vi "typedef test.vi"() -> ()   [LabVIEW 2023]
uses:
  JSON Schema Generator.lvlib
  <vilib>/JDP Science/JSONtext/JSONtext.lvlib
  Example/Example Cluster 1.ctl
panel:
  out "error out":errorcluster
  in  "Example Cluster":T1={"ProductId"=1, "productName"="A green door", "price"=12.5, "tags"=["home", "green"], "ProductNumber"=1, "ProductInfoInternal"={"ProductState"=enum."Active", "State Info"={"Date"="", "Time"=0.0}}, "Product History"=[]}
  out "<JSON>":string
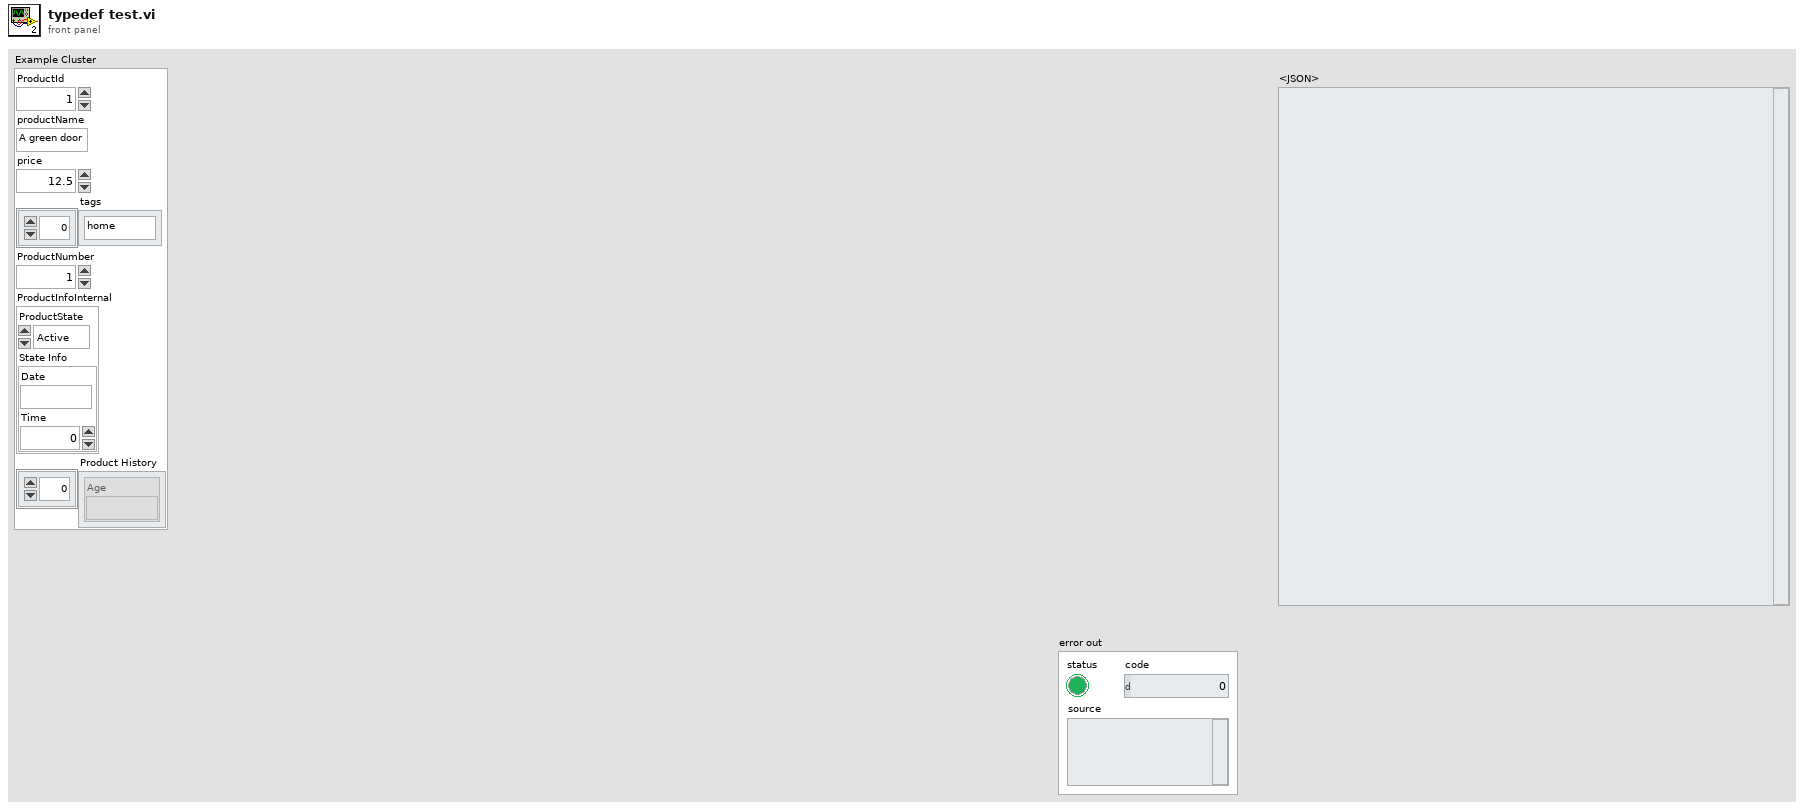
[diagram p1: front panel]
types:
  T1 = typedef "Example Cluster 1.ctl" = cluster{"ProductId":i32, "productName":string, "price":dbl, "tags":string[], "ProductNumber":i32, "ProductInfoInternal":cluster{"ProductState":enum16{"Active", "InActive"}, "State Info":cluster{"Date":string, "Time":dbl}}, "Product History":cluster{"Age":string}[]}
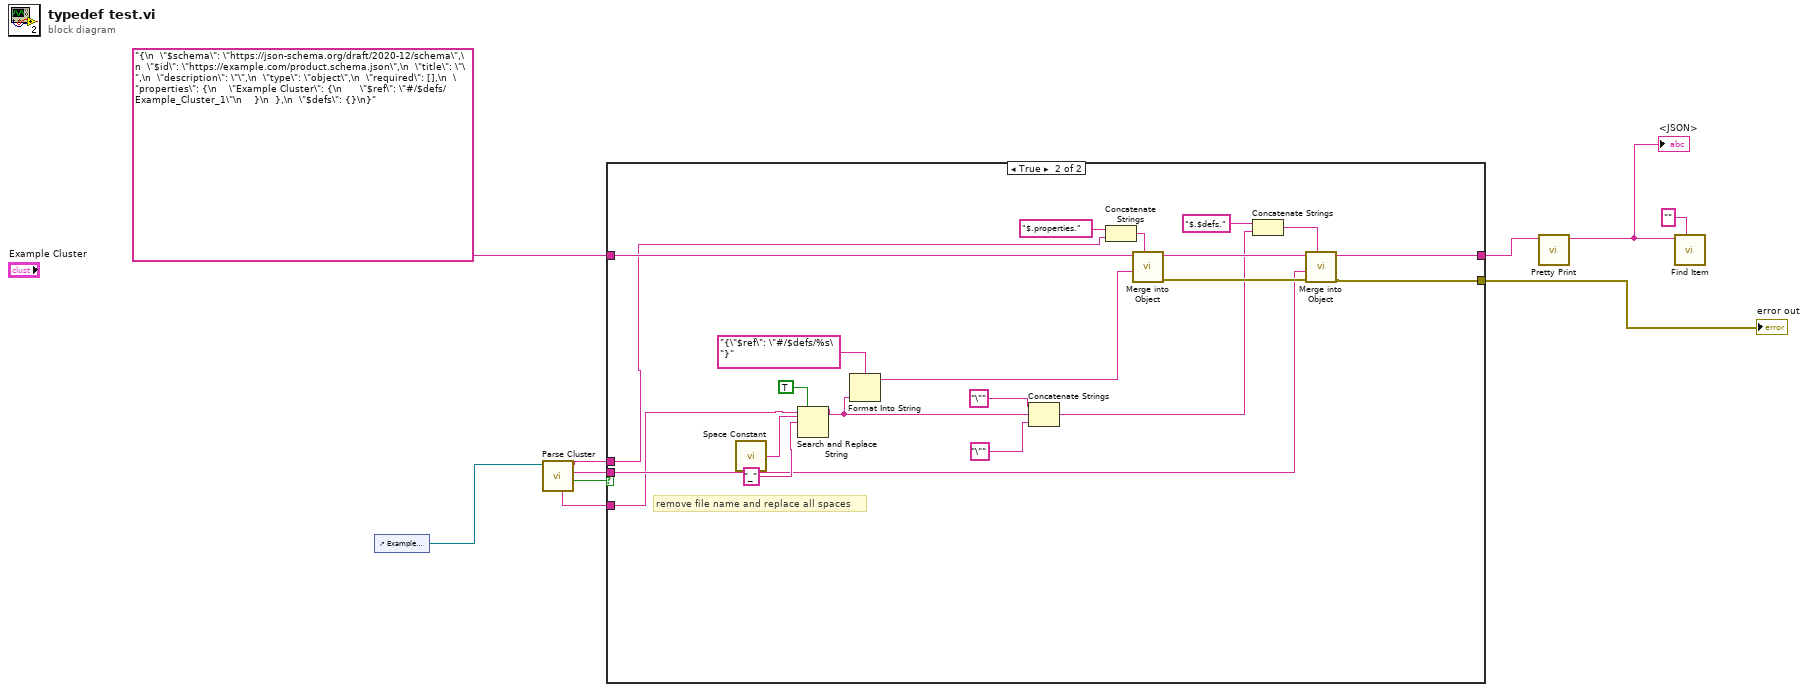
[diagram p0: block diagram]
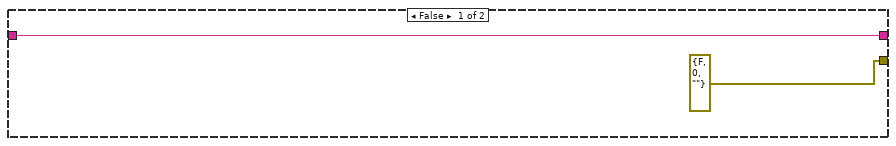
[diagram p2: hidden frame]
diagram:
  n1 = control-ref of="Example Cluster"() -> (w7:refnum<vi>)
  n2 = call "Parse Cluster.vi"("Cluster Refnum In"=w7) -> ("Typedef?"=w3:bool, "JSON ObjectSchema out"=w6:string, "JSON Object Name"=w1:string, "Typedef Name"=w2:string)  [unwired: 6 in, 1 out]
  n3 = case shown="True" w3 {
    tunnel: [w11 w29] -> w10
    tunnel: [errorcluster {"status"=FALSE, "code"=0, "source"=""} ("error out") w24] -> w9
    tunnel: "{\n  \"$schema\": \"https://json-schema.org/draft/2020-12/schema\",\n  \"$id\": \"https://example.com/product.schema.json\",\n  \"title\": \"\",\n  \"description\": \"\",\n  \"type\": \"object\",\n  \"required\": [],\n  \"properties\": {\n    \"Example Cluster\": {\n      \"$ref\": \"#/$defs/Example_Cluster_1\"\n    }\n  },\n  \"$defs\": {}\n}" ("JSON") -> [w11 w19]
    tunnel: w6 -> [_ w18]
    tunnel: w2 -> [_ w14]
    tunnel: w1 -> [_ w13]
    frame False {
    }
    frame True {
      # "remove file name and replace all spaces"
      n4 = call <vilib>:"Space Constant.vi"() -> ("String"=w21:string)
      n5 = Search and Replace String(replace all?=TRUE ("replace all? (F)"), input string=w14, search string=w21, replace string="_" ("replace string (\"\")")) -> (result string=w23:string)  [unwired: 4 in, 3 out]
      n6 = Format Into String(format string="{\"$ref\": \"#/$defs/%s\"}", w23) -> (resulting string=w26:string)  [unwired: 2 in, 1 out]
      n7 = Concatenate Strings("\"" ("string"), w23, "\"" ("string")) -> (w17:string)
      n8 = Concatenate Strings("$.properties." ("$Path or Item Name"), w13) -> (w32:string)
      n9 = call <vilib>:"Merge into Object.vi"("$Path or Item Name"=w32, "JSON Object to Merge"=w26, "JSON"=w19) -> ("error out"=w25:errorcluster, "<JSON>"=w30:string)  [unwired: 6 in]
      n10 = Concatenate Strings("$.$defs." ("$Path or Item Name"), w17) -> (w27:string)
      n11 = call <vilib>:"Merge into Object.vi"("$Path or Item Name"=w27, "error in (no error)"=w25, "JSON Object to Merge"=w18, "JSON"=w30) -> ("error out"=w24:errorcluster, "<JSON>"=w29:string)  [unwired: 5 in]
    }
  }
  "error out" <- w9
  n12 = call <vilib>:"Pretty Print.vi"("JSON"=w10) -> ("<JSON>"=w5:string)  [unwired: 8 in, 2 out]
  "<JSON>" <- w5
  n13 = call <vilib>:"Find Item.vi"("$Path or Item Name"="", "JSON"=w5) -> ()  [unwired: 6 in, 4 out]
